vi "Begin.vi"(8 "error in":errorcluster) -> (0 "error out":errorcluster)   [LabVIEW 2020]
doc: "Called before other user functions, this VI is expected to open initial I/O refnums, load in file data, and do all program initialization. Notice that the <B>error out</B> terminal is simply used for data flow. Wiring it to other structures or subVIs ensures that this VI runs first."
uses:
  <vilib>/Rock Robotics/WPI/DriverStation/WPI_DriverStationRobotMode2.ctl
  <vilib>/Rock Robotics/WPI/Joystick/WPI_JoystickDeviceEnum.ctl
  Robot Global Data.vi
  <vilib>/Rock Robotics/WPI/ThirdParty/Phoenix-LabVIEW/Pigeon IMU/CTRE_PigeonIMU_Open_CAN.vi
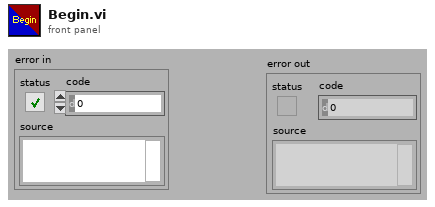
[diagram p1: front panel]
types:
  T1 = typedef "WPI_JoystickDeviceEnum.ctl" = enum16{"USB 0", "USB 1", "USB 2", "USB 3", "USB 4", "USB 5"}
  T2 = typedef "WPI_DriverStationRobotMode2.ctl" = enum16{"Autonomous Disabled", "Autonomous Enabled", "Teleop Disabled", "Teleop Enabled", "Disconnected", "Finish", "Test Disabled", "Test Enabled", "Emergency Stopped"}
  T3 = typedef "WPI_JoystickDevRef.ctl" = cluster{"Device":T1}
  T4 = typedef "CTRE_PigeonIMU_DeviceRef.ctl" = cluster{"DeviceStatus":errorcluster, "Device Number":u8, "Type":T5, "Device ID":u32, "Handle":u64, "UsageFrame":u32, "Library Path":path}
  T5 = typedef "CTRE_PigeonIMU_ConnectionType.ctl" = u32
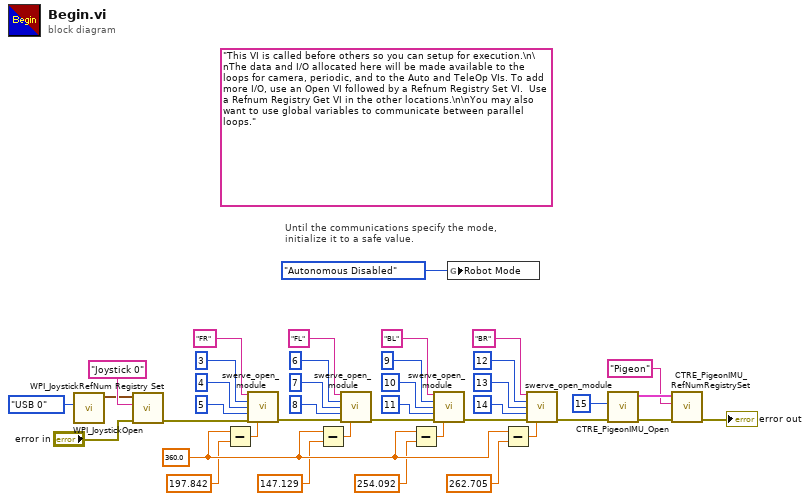
[diagram p0: block diagram]
diagram:
  w5 = 360.0 ("Encoder Offset (Deg)")
  (unwired) "This VI is called before others so you can setup for execution.\n\nThe data and I/O allocated here will be made available to the loops for camera, periodic, and to the Auto and TeleOp VIs. To add more I/O, use an Open VI followed by a Refnum Registry Set VI.  Use a Refnum Registry Get VI in the other locations.\n\nYou may also want to use global variables to communicate between parallel loops."
  # "Until the communications specify the mode,\ninitialize it to a safe value."
  n1 = call <vilib>:"WPI_JoystickOpen.vi"("JoystickDevice"=WPI_JoystickDeviceEnum."USB 0") -> ("JoystickDevRef"=w38:T3)  [unwired: 10 in]
  n2 = call <vilib>:"WPI_JoystickRefNum Registry Set.vi"("error in (no error)"="error in", "refnum name"="Joystick 0", "JoystickDevRef"=w38) -> ("error out"=w12:errorcluster)  [unwired: 7 in, 1 out]
  n3 = Subtract(x=w5, y=197.842 ("Encoder Offset (Deg)")) -> (x-y=w9:dbl)
  n4 = call "swerve_open_module.vi"("Module Suffix"="FR", "Drive CAN ID"=u8 3, "Azimuth CAN ID"=u8 4 ("Drive CAN ID"), "Encoder CAN ID"=u8 5 ("Drive CAN ID"), "error in"=w12, "Encoder Offset (Deg)"=w9) -> ("error out"=w24:errorcluster)  [unwired: 9 in]
  n5 = Subtract(x=w5, y=147.129 ("Encoder Offset (Deg)")) -> (x-y=w8:dbl)
  n6 = call "swerve_open_module.vi"("Module Suffix"="FL", "Drive CAN ID"=u8 6, "Azimuth CAN ID"=u8 7 ("Drive CAN ID"), "Encoder CAN ID"=u8 8 ("Drive CAN ID"), "error in"=w24, "Encoder Offset (Deg)"=w8) -> ("error out"=w19:errorcluster)  [unwired: 9 in]
  n7 = Subtract(x=w5, y=254.092 ("Encoder Offset (Deg)")) -> (x-y=w7:dbl)
  n8 = call "swerve_open_module.vi"("Module Suffix"="BL", "Drive CAN ID"=u8 9, "Azimuth CAN ID"=u8 10 ("Drive CAN ID"), "Encoder CAN ID"=u8 11 ("Drive CAN ID"), "error in"=w19, "Encoder Offset (Deg)"=w7) -> ("error out"=w14:errorcluster)  [unwired: 9 in]
  n9 = global write "Robot Global Data.vi" "Robot Mode"(WPI_DriverStationRobotMode2."Autonomous Disabled" ("Robot Mode")) -> ()
  n10 = Subtract(x=w5, y=262.705 ("Encoder Offset (Deg)")) -> (x-y=w6:dbl)
  n11 = call "swerve_open_module.vi"("Module Suffix"="BR", "Drive CAN ID"=u8 12, "Azimuth CAN ID"=u8 13 ("Drive CAN ID"), "Encoder CAN ID"=u8 14 ("Drive CAN ID"), "error in"=w14, "Encoder Offset (Deg)"=w6) -> ("error out"=w11:errorcluster)  [unwired: 9 in]
  n12 = call-poly <vilib>:"CTRE_PigeonIMU_Open.vi"("error in"=w11, "Device Number"=u8 15) -> ("error out"=w35:errorcluster, "PigeonIMUDevRef"=w34:T4)  [unwired: 8 in]
  n13 = call <vilib>:"CTRE_PigeonIMU_RefNumRegistrySet.vi"("error in (no error)"=w35, "refnum name"="Pigeon", "PigeonIMUDevRef"=w34) -> ("error out"=→"error out":errorcluster)  [unwired: 7 in, 1 out]
